vi "Get Test Name.vi"(2 "id number":u32, 3 "which board":T1) -> (0 "test name":string)   [LabVIEW 2018]
doc: "Build a test name from the board type and the identification number."
uses:
  Common/Board Type Enum.ctl
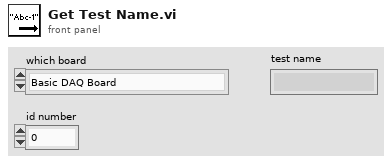
[diagram p1: front panel]
types:
  T1 = typedef "Board Type Enum.ctl" = enum16{"Basic DAQ Board", "Elite DAQ Board", "GPIB Board"}
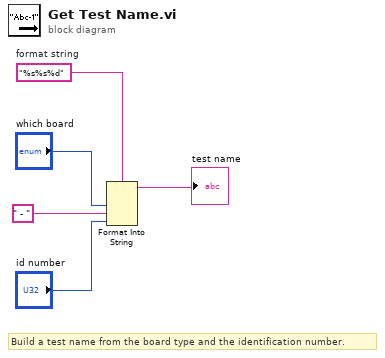
[diagram p0: block diagram]
diagram:
  w5 = "%s%s%d"  # format string
  # "Build a test name from the board type and the identification number."
  n1 = Format Into String(format string=w5, "which board", " - ", "id number") -> (resulting string=→"test name":string)  [unwired: 2 in, 1 out]
